vi "Open Spreadsheet.vi"(6 "Version (Excel 2007+)":enum16{"Excel 2007+", "Excel 2003-"}(ring), 7 "Create if does not exist? (T)":bool=TRUE, 8 "error in (no error)":errorcluster, 10 "File Name":path) -> (0 "error out":errorcluster, 3 "Spreadsheet":refnum<class "Spreadsheet.lvclass">)   [LabVIEW 2013, in "Spreadsheet.lvclass"]
uses:
  OOP/Spreadsheet.lvclass
  OOP/Excel Legacy/Excel Legacy.lvclass
  OOP/Excel XML/Excel XML.lvclass
  OOP/Spreadsheet.lvclass/Spreadsheet.ctl
  <vilib>/Utility/error.llb/Error Cluster From Error Code.vi
  <vilib>/ErrorRing/Error Ring.xnode
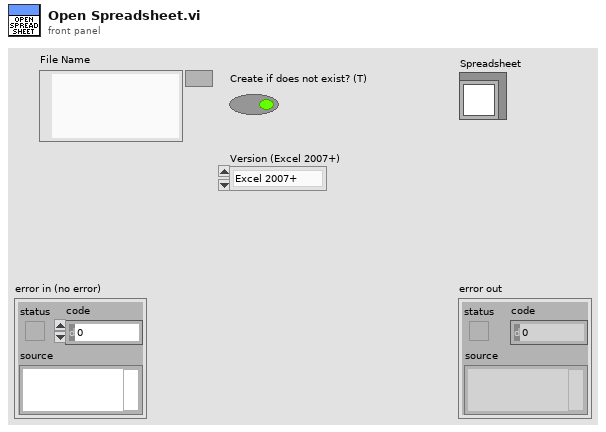
[diagram p1: front panel]
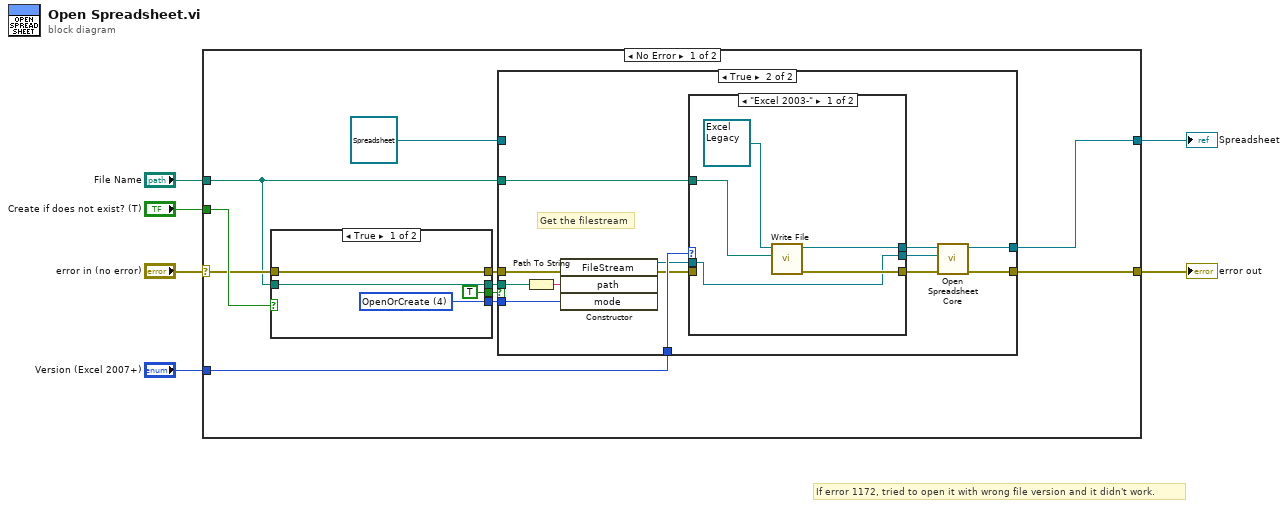
[diagram p0: block diagram]
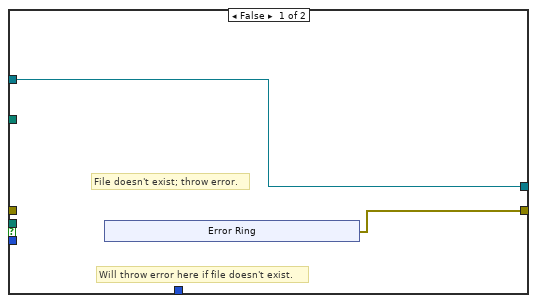
[diagram p2: hidden frame]
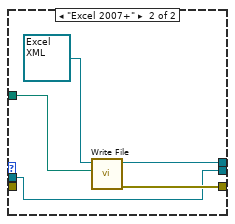
[diagram p3: hidden frame]
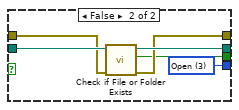
[diagram p4: hidden frame]
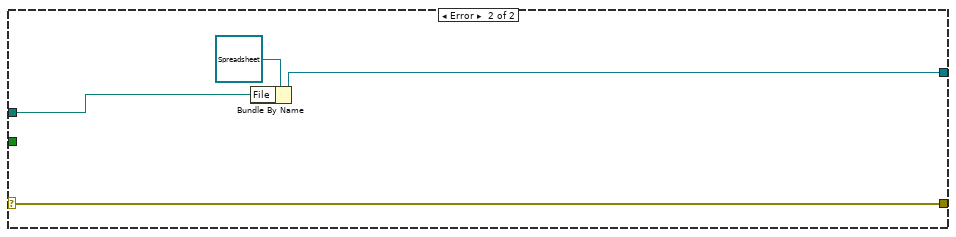
[diagram p5: hidden frame]
diagram:
  # "If error 1172, tried to open it with wrong file version and it didn't work."
  n1 = case shown="No Error" "error in (no error)" {
    selector: "error in (no error)" -> [w12 w60]
    tunnel: [w9 w60] -> w5
    tunnel: [w10 w59] -> w1
    tunnel: "File Name" -> [w8 w58]
    tunnel: "Create if does not exist? (T)" -> [w13 _]
    tunnel: "Version (Excel 2007+)" -> [w11 _]
    frame No Error {
      n2 = case shown="True" w13 {
        tunnel: [w50 w56] -> w14
        tunnel: [w49 w52] -> w15
        tunnel: w12 -> [w49 w53]
        tunnel: [w48 w54] -> w16
        tunnel: w8 -> [w48 w55]
        tunnel: [TRUE ("file or folder exists?") w51] -> w17
        frame True {
          w50 = 4 items=["CreateNew"=1, "Create"=2, "Open"=3, "OpenOrCreate"=4, "Truncate"=5, "Append"=6] ("mode")
        }
        frame False {
          w56 = 3 items=["CreateNew"=1, "Create"=2, "Open"=3, "OpenOrCreate"=4, "Truncate"=5, "Append"=6] ("mode")
          n3 = call <vilib>:"Check if File or Folder Exists.vi"("error in (no error)"=w53, "path"=w55) -> ("error out"=w52:errorcluster, "file or folder exists?"=w51:bool, "dup path"=w54:path)  [unwired: 7 in]
        }
      }
      n4 = case shown="True" w17 {
        tunnel: w14 -> [_ w33]
        tunnel: w15 -> [_ w34]
        tunnel: w16 -> [_ w32]
        tunnel: w11 -> [_ w36]
        tunnel: [w18 w26] -> w10
        tunnel: [w19 w28] -> w9
        tunnel: w8 -> [_ w24]
        tunnel: refnum<class "Spreadsheet.lvclass"> refnum ("Spreadsheet.lvclass") -> [w18 _]
        frame False {
          # "File doesn't exist; throw error."
          # "Will throw error here if file doesn't exist."
          n5 = xnode "Error Ring"() -> ("error out"=w19:errorcluster)
        }
        frame True {
          # "Get the filestream"
          n6 = Path To String(path=w32) -> (string=w35:string)
          n7 = constructor class="FileStream"(error in=w34, "path"=w35, "mode"=w33) -> (reference out=w30:refnum<k24>, error out=w31:errorcluster)  [unwired: 2 in, 3 out]
          n8 = case shown="\"Excel 2003-\"" w36 {
            tunnel: [w38 w44] -> w27
            tunnel: w31 -> [_ _]
            tunnel: w30 -> [w37 w43]
            tunnel: [w40 w46] -> w29
            tunnel: [w37 w43] -> w25
            tunnel: w24 -> [w39 w45]
            frame "Excel 2003-" {
              n9 = call-dynamic "Write File.vi"("File"=w39, "Spreadsheet in"=refnum<class "Excel Legacy.lvclass"> refnum ("Excel Legacy.lvclass")) -> ("error out"=w40:errorcluster, "Spreadsheet out"=w38:refnum<class "Excel Legacy.lvclass">)  [unwired: 8 in]
            }
            frame "Excel 2007+" {
              n10 = call-dynamic "Write File.vi"("File"=w45, "Spreadsheet in"=refnum<class "Excel XML.lvclass"> refnum ("Excel XML.lvclass")) -> ("error out"=w46:errorcluster, "Spreadsheet out"=w44:refnum<class "Excel XML.lvclass">)  [unwired: 8 in]
            }
          }
          n11 = call-dynamic "Open Spreadsheet Core.vi"("error in (no error)"=w29, "FileStream"=w25, "Spreadsheet in"=w27) -> ("error out"=w28:errorcluster, "Spreadsheet out"=w26:refnum<class "Spreadsheet.lvclass">)  [unwired: 7 in]
        }
      }
    }
    frame Error {
      n12 = Bundle By Name(cluster=refnum<class "Spreadsheet.lvclass"> refnum ("Spreadsheet.lvclass"), "File"=w58) -> (w59:refnum<class "Spreadsheet.lvclass">)
    }
  }
  "error out" <- w5
  "Spreadsheet" <- w1
